vi "Terminal_Global_Template_Name.vi"() -> ()   [LabVIEW 2014]
panel:
  out "模板名称":string
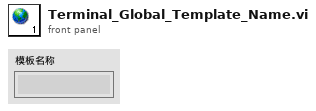
[diagram p1: front panel]
diagram:
